vi "op_biti_v6.vi"() -> ()   [LabVIEW 2010]
panel:
  out "L0":bool=TRUE
  out "L1":bool
  out "L2":bool=TRUE
  out "L3":bool
  out "L4":bool=TRUE
  out "L5":bool
  out "L6":bool=TRUE
  out "L7":bool
  in  "K0":bool=TRUE
  in  "K1":bool
  in  "K2":bool=TRUE
  in  "K3":bool
  in  "K4":bool=TRUE
  in  "K5":bool
  in  "K6":bool=TRUE
  in  "K7":bool
  out "Numeric":dbl=85.0
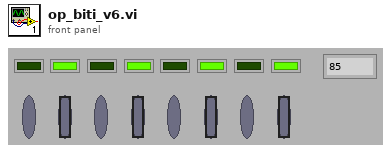
[diagram p1: front panel]
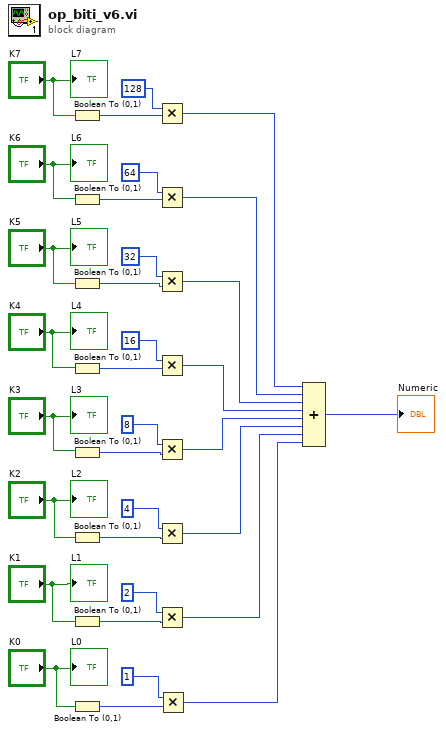
[diagram p0: block diagram]
diagram:
  n1 = Boolean To (0,1)(Boolean="K7") -> (0, 1=w32:i16)
  n2 = Boolean To (0,1)(Boolean="K6") -> (0, 1=w30:i16)
  n3 = Boolean To (0,1)(Boolean="K5") -> (0, 1=w29:i16)
  n4 = Boolean To (0,1)(Boolean="K4") -> (0, 1=w28:i16)
  n5 = Boolean To (0,1)(Boolean="K3") -> (0, 1=w27:i16)
  n6 = Boolean To (0,1)(Boolean="K2") -> (0, 1=w26:i16)
  n7 = Boolean To (0,1)(Boolean="K1") -> (0, 1=w25:i16)
  n8 = Boolean To (0,1)(Boolean="K0") -> (0, 1=w24:i16)
  n9 = Multiply(x=128, y=w32) -> (x*y=w9:i32)
  n10 = Multiply(x=64, y=w30) -> (x*y=w8:i32)
  n11 = Multiply(x=32, y=w29) -> (x*y=w7:i32)
  n12 = Multiply(x=16, y=w28) -> (x*y=w6:i32)
  n13 = Multiply(x=8, y=w27) -> (x*y=w5:i32)
  n14 = Multiply(x=4, y=w26) -> (x*y=w4:i32)
  n15 = Multiply(x=2, y=w25) -> (x*y=w3:i32)
  n16 = Multiply(x=1, y=w24) -> (x*y=w2:i32)
  n17 = Compound Arithmetic op=ADD(w9, w8, w7, w6, w5, w4, w3, w2) -> (→"Numeric":i32)
  "L7" <- "K7"
  "L6" <- "K6"
  "L5" <- "K5"
  "L4" <- "K4"
  "L3" <- "K3"
  "L2" <- "K2"
  "L1" <- "K1"
  "L0" <- "K0"
